vi "Rpt _Get _PCBARepair.vi"(5 "IntSN":string, 6 "DateTo":string, 7 "DateFrom":string, 8 "error in (no error)":errorcluster caption="错误输入（无错误）", 9 "Model":string, 10 "prodorder":string, 11 "Traceability 引用句柄":refnum<k24>) -> (0 "error out":errorcluster caption="错误输出", 2 ".NET:System.Data.DataSet":T1={"CaseSensitive"=FALSE, "Container"=refnum, "DataSetName"="", "DefaultViewManager"=refnum, "DesignMode"=FALSE, "EnforceConstraints"=FALSE, "ExtendedProperties"=refnum, "HasErrors"=FALSE, "IsInitialized"=FALSE, "Locale"=refnum, "Namespace"="", "Prefix"="", "Relations"=refnum, "RemotingFormat"=0, "SchemaSerializationMode"=1, "Site"=refnum, "Tables"=refnum} {"SchemaSerializationMode" items=["IncludeSchema"=1, "ExcludeSchema"=2]; "RemotingFormat" items=["Xml", "Binary"]}, 3 "Traceability 引用句柄输出":refnum<k24>)   [LabVIEW 2014, in "Traceability.lvlib"]
uses:
  D:/webservice/Traceability.dll
  Traceability.dll
  System.Data
  Traceability.lvlib
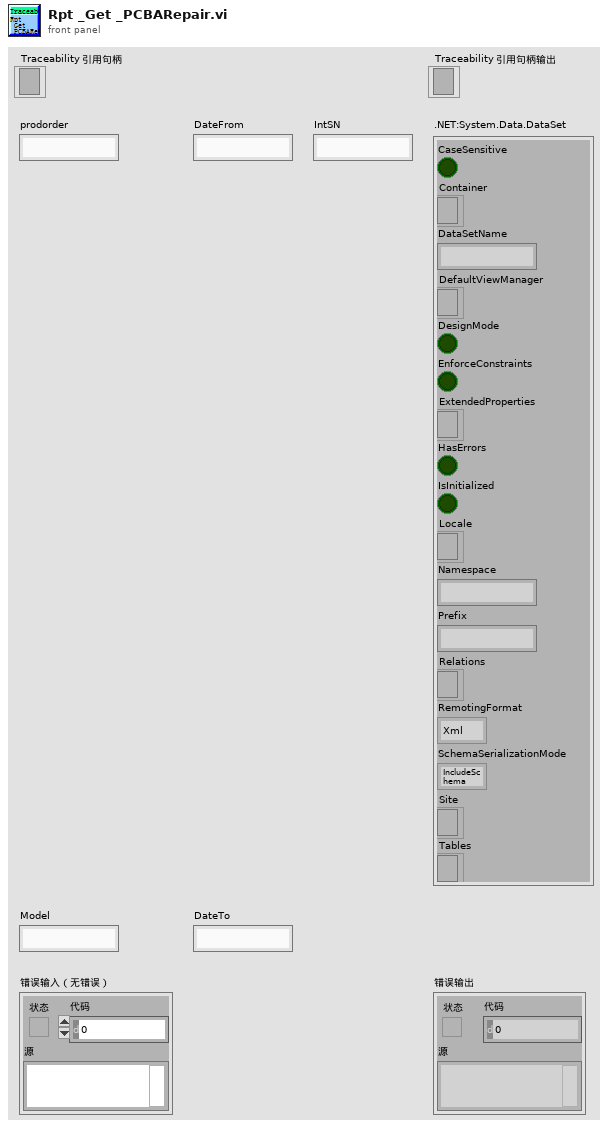
[diagram p1: front panel]
types:
  T1 = cluster{"CaseSensitive":bool, "Container":refnum<k24>, "DataSetName":string, "DefaultViewManager":refnum<k24>, "DesignMode":bool, "EnforceConstraints":bool, "ExtendedProperties":refnum<k24>, "HasErrors":bool, "IsInitialized":bool, "Locale":refnum<k24>, "Namespace":string, "Prefix":string, "Relations":refnum<k24>, "RemotingFormat":i32, "SchemaSerializationMode":i32, "Site":refnum<k24>, "Tables":refnum<k24>}
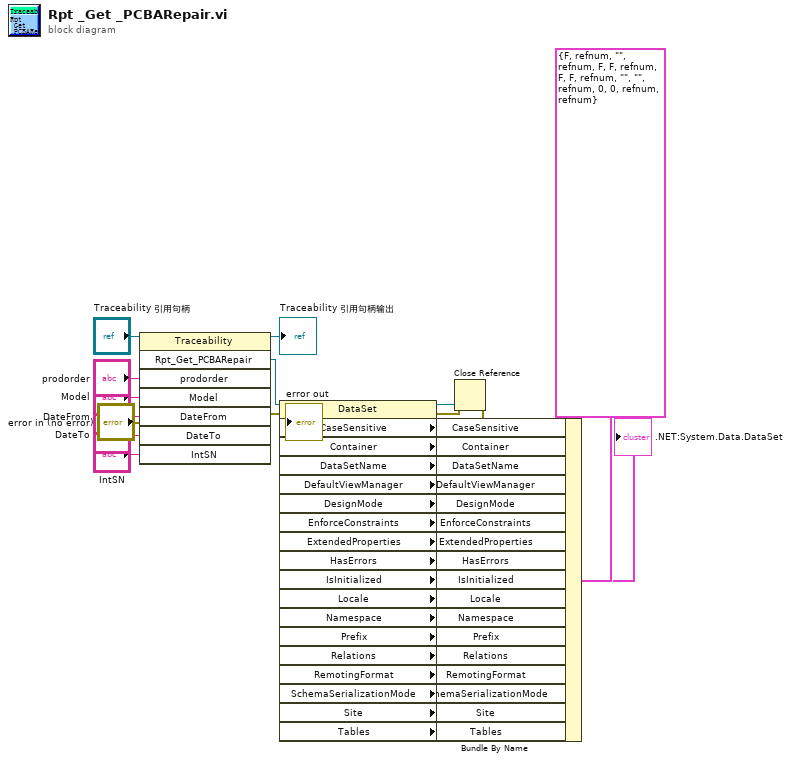
[diagram p0: block diagram]
diagram:
  n1 = invoke class="Traceability" method="Rpt_Get_PCBARepair"(reference="Traceability 引用句柄", error in="error in (no error)", "prodorder"="prodorder", "Model"="Model", "DateFrom"="DateFrom", "DateTo"="DateTo", "IntSN"="IntSN") -> (reference out=→"Traceability 引用句柄输出":refnum<k24>, error out=w4:errorcluster, "Rpt_Get_PCBARepair"=w29:refnum<k24>)  [unwired: 1 in, 5 out]
  n2 = property class="DataSet"(reference=w29, error in=w4) -> (reference out=w3:refnum<k24>, error out=w2:errorcluster, "CaseSensitive"=w26:bool, "Container"=w25:refnum<k24>, "DataSetName"=w24:string, "DefaultViewManager"=w23:refnum<k24>, "DesignMode"=w22:bool, "EnforceConstraints"=w21:bool, "ExtendedProperties"=w20:refnum<k24>, "HasErrors"=w19:bool, "IsInitialized"=w18:bool, "Locale"=w17:refnum<k24>, "Namespace"=w16:string, "Prefix"=w15:string, "Relations"=w14:refnum<k24>, "RemotingFormat"=w13:i32, "SchemaSerializationMode"=w12:i32, "Site"=w11:refnum<k24>, "Tables"=w10:refnum<k24>)
  n3 = Bundle By Name(cluster=T1 {"CaseSensitive"=FALSE, "Container"=refnum, "DataSetName"="", "DefaultViewManager"=refnum, "DesignMode"=FALSE, "EnforceConstraints"=FALSE, "ExtendedProperties"=refnum, "HasErrors"=FALSE, "IsInitialized"=FALSE, "Locale"=refnum, "Namespace"="", "Prefix"="", "Relations"=refnum, "RemotingFormat"=0, "SchemaSerializationMode"=0, "Site"=refnum, "Tables"=refnum} (".NET:System.Data.DataSet"), "CaseSensitive"=w26, "Container"=w25, "DataSetName"=w24, "DefaultViewManager"=w23, "DesignMode"=w22, "EnforceConstraints"=w21, "ExtendedProperties"=w20, "HasErrors"=w19, "IsInitialized"=w18, "Locale"=w17, "Namespace"=w16, "Prefix"=w15, "Relations"=w14, "RemotingFormat"=w13, "SchemaSerializationMode"=w12, "Site"=w11, "Tables"=w10) -> (→".NET:System.Data.DataSet":T1)
  n4 = Close Reference(reference=w3, error in (no error)=w2) -> (error out=→"error out":errorcluster)
